vi "Do.vi"(8 "error in":errorcluster, 10 "Actor in":refnum<class "Actor.lvclass">, 11 "Change Red Laser DC MSG":refnum<class "Change Red DC MSG.lvclass">) -> (0 "error out":errorcluster, 2 "Actor out":refnum<class "Actor.lvclass">)   [LabVIEW 2014, in "eCRDS Library.lvlib" / "Change Red DC MSG.lvclass"]
doc: "(<B>Filename</B>: Actor Framework.lvlib:Message.lvclass:Do.vi)\n\nDefines what a message does when it is received by an actor. Generally, a message instructs an actor to invoke one of its methods. By default, this method does nothing. A child class must override it to define behavior. Create a child class by using the Actor Framework Message Maker dialog box."
uses:
  Change Red DC MSG.lvclass
  <vilib>/ActorFramework/Actor/Actor.lvclass
  Change Red DC MSG.lvclass/Change Red DC MSG.ctl
  Instr Actor/Instr Actor.lvclass
  Commands/Update Red DC/Update Red DC.lvclass
  Commands/Update Red DC/Update Red DC.lvclass/Update Red DC.ctl
  SuperActor/SuperActor.lvclass/SuperActor.ctl
  SuperActor/Read CVT Session.vi
  SuperActor/Read Log Session.vi
  <userlib>/_Session Fwk/Session - Root.lvclass
  reusable/Command/Command.lvclass
  reusable/Session APIs/Session Log/System Log.lvclass
  reusable/Session APIs/CVT/CVT.lvclass
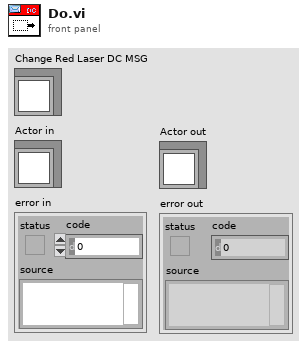
[diagram p1: front panel]
types:
  T1 = typedef "Session - Root.lvclass/Session Handle.ctl" = refnum<data-value>
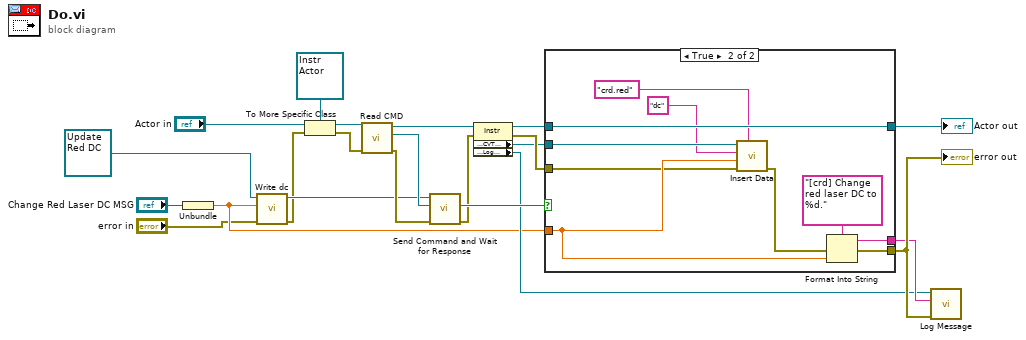
[diagram p0: block diagram]
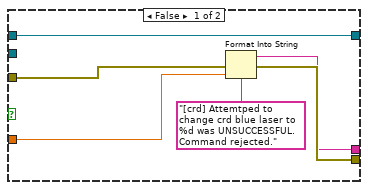
[diagram p2: hidden frame]
diagram:
  n1 = Unbundle("Change Red Laser DC MSG") -> (w3:dbl)
  n2 = call "Write dc.vi"("error in (no error)"="error in", "dc"=w3, "Update Blue DC in"=refnum<class "Update Red DC.lvclass"> refnum ("eCRDS Library.lvlib: Update Red DC.lvclass")) -> ("error out"=w1:errorcluster, "Update Blue DC out"=w4:refnum<class "Update Red DC.lvclass">)  [unwired: 7 in]
  n3 = To More Specific Class(target class=refnum<class "Instr Actor.lvclass"> refnum ("Instrument Lib:Instr"), reference="Actor in", error in=w1) -> (specific class reference=w20:refnum<class "Instr Actor.lvclass">, error out=w18:errorcluster)
  n4 = call "Read CMD.vi"("error in (no error)"=w18, "Instr Actor in"=w20) -> ("error out"=w16:errorcluster, "CMD"=w17:refnum<queue>, "Instr Actor out"=w13:refnum<class "Instr Actor.lvclass">)  [unwired: 7 in]
  n5 = call "Send Command and Wait for Response.vi"("error in"=w16, "cmd queue"=w17, "CMD in"=w4) -> ("error out"=w11:errorcluster, "cmd good?"=w15:bool)  [unwired: 6 in, 1 out]
  n6 = property class="Instr"(reference=w13, error in=w11) -> (reference out=w12:refnum<class "Instr Actor.lvclass">, error out=w9:errorcluster, "Accessors:CVT Session"=w6:T1, "Accessors:Log Session"=w7:T1)
  n7 = case shown="True" w15 {
    tunnel: w3 -> [w27 w31]
    tunnel: w12 -> [w28 w38]
    tunnel: [w28 w38] -> w14
    tunnel: w9 -> [w25 w30]
    tunnel: [w24 w35] -> w10
    tunnel: [w23 w36] -> w8
    tunnel: w6 -> [_ w33]
    frame False {
      n8 = Format Into String(format string="[crd] Attemtped to change crd blue laser to %d was UNSUCCESSFUL.  Command rejected.", error in=w25, w27) -> (resulting string=w23:string, error out=w24:errorcluster)  [unwired: 1 in]
    }
    frame True {
      n9 = call "Insert Data.vi"("Group"="crd.red", "error in"=w30, "Data"=w31, "tag"="dc", "CVT Session In"=w33) -> ("error out"=w29:errorcluster)  [unwired: 5 in, 1 out]
      n10 = Format Into String(format string="[crd] Change red laser DC to %d.", error in=w29, w31) -> (resulting string=w36:string, error out=w35:errorcluster)  [unwired: 1 in]
    }
  }
  "error out" <- w10
  "Actor out" <- w14
  n11 = call "Log Message.vi"("error in"=w10, "MSG In"=w8, "session in"=w7) -> ()  [unwired: 7 in, 2 out]
